vi "Save Rectifier Recipe.vi"(5 "Rev Mult":dbl format="%#_13g", 6 "Right AmpMins":dbl[](array[numeric]), 7 "Left AmpMins":dbl[](array[numeric]), 8 "error in":errorcluster, 9 "Number Steps":i32, 10 "Right Amps":dbl[](array[numeric]), 11 "Left Amps":dbl[](array[numeric])) -> (0 "error out":errorcluster, 2 "name":string, 3 "cancelled":bool)   [LabVIEW 2019]
uses:
  <vilib>/Utility/sysdir.llb/System Directory Type.ctl
  <vilib>/Utility/config.llb/Write Key (I32).vi
  <vilib>/Utility/config.llb/Write Key (Double).vi
  <vilib>/Utility/config.llb/NI_LVConfig.lvlib
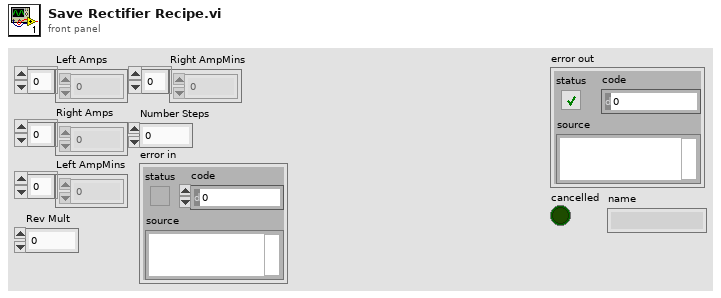
[diagram p1: front panel]
types:
  T1 = typedef "System Directory Type.ctl" = i32
  T2 = typedef "NI_LVConfig.lvlib/Config Data RefNum.ctl" = refnum<k1>
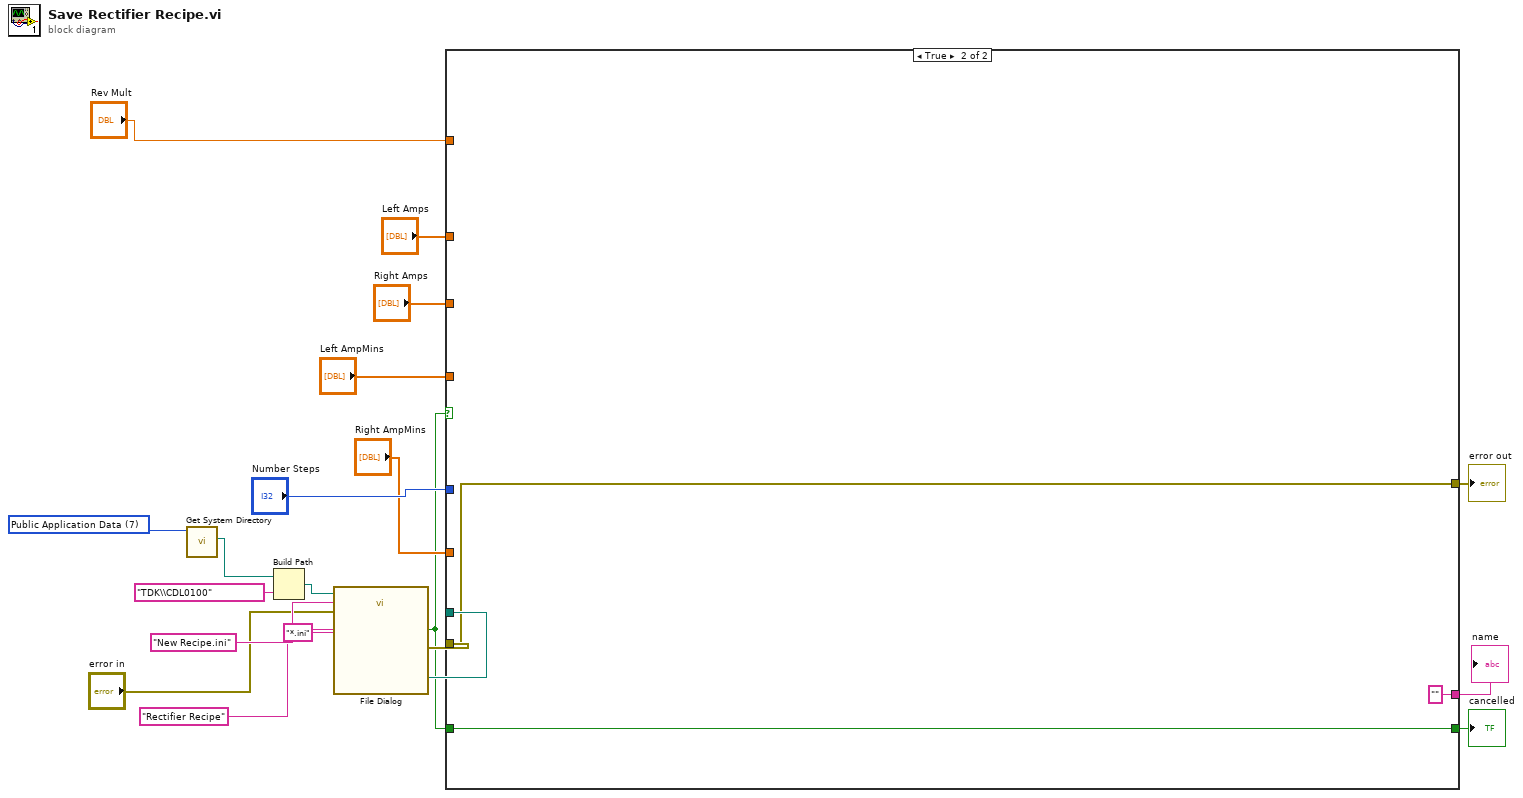
[diagram p0: block diagram]
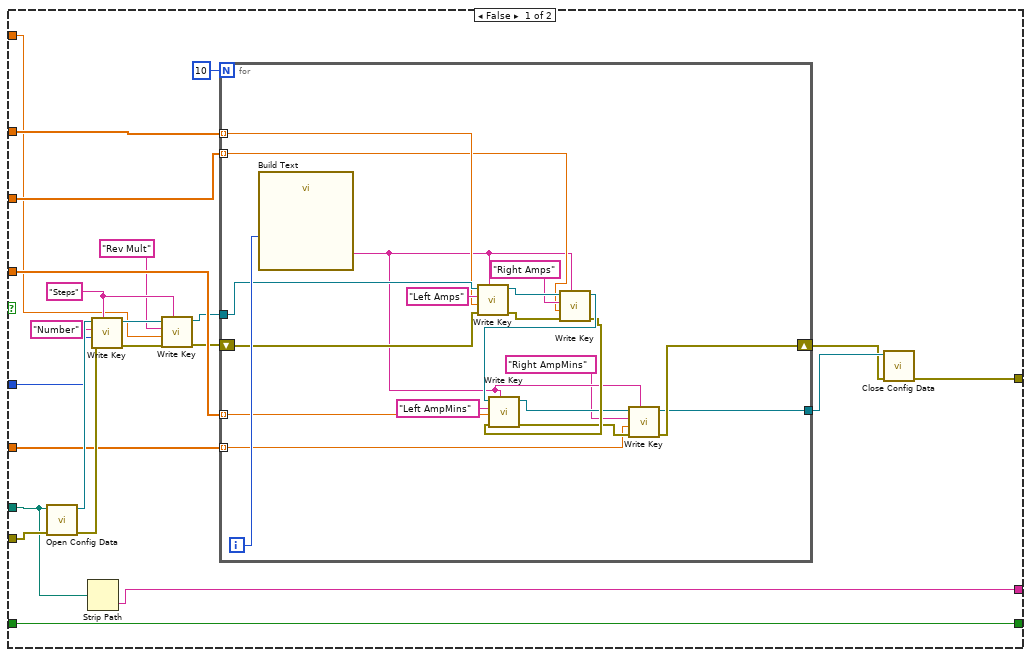
[diagram p2: hidden frame]
diagram:
  w20 = T1 7 items=["User Home"=0, "User Desktop"=1, "User Documents"=2, "User Application Data"=3, "User Preferences"=4, "User Temporary"=5, "Public Documents"=6, "Public Application Data"=7, "Public Preferences"=8, "Public Cache"=13, "System Core Libraries"=9, "System Installed Libraries"=10, "Application Files"=11, "Boot Volume Root"=12] ("system directory type")
  n1 = call <vilib>:"Get System Directory.vi"("system directory type"=w20) -> ("system directory"=w19:path)  [unwired: 10 in]
  n2 = Build Path(base path=w19, name or relative path="TDK\\CDL0100") -> (appended path=w17:path)
  n3 = call "File Dialog"("start path"=w17, "default name"="New Recipe.ini", "error in"="error in", "pattern (all files)"="*.ini", "pattern label"="Rectifier Recipe") -> ("selected path"=w12:path, "cancelled"=w3:bool, "error out"=w11:errorcluster)  [unwired: 7 in, 1 out]
  n4 = case shown="True" w3 {
    tunnel: w12 -> [w23 _]
    tunnel: w11 -> [w42 w66]
    tunnel: "Number Steps" -> [w39 _]
    tunnel: "Left Amps" -> [w37 _]
    tunnel: "Right Amps" -> [w36 _]
    tunnel: "Left AmpMins" -> [w35 _]
    tunnel: "Right AmpMins" -> [w34 _]
    tunnel: [w31 w66] -> w5
    tunnel: "Rev Mult" -> [w24 _]
    tunnel: w3 -> [w22 w65]
    tunnel: [w22 w65] -> w2
    tunnel: [w21 "" ("name")] -> w1
    frame False {
      w28 = "Steps" ("section")
      n5 = call <vilib>:"Open Config Data.vi"("error in (no error)"=w42, "configuration file path"=w23) -> ("error out"=w38:errorcluster, "refnum"=w41:T2)  [unwired: 7 in, 1 out]
      n6 = Strip Path(path=w23) -> (name=w21:string)  [unwired: 1 out]
      n7 = call-poly <vilib>:"Write Key.vi"("section"=w28, "error in (no error)"=w38, "value"=w39, "key"="Number", "refnum"=w41) -> ("error out"=w27:errorcluster, "refnum out"=w30:T2)  [unwired: 4 in, 1 out]
      n8 = call-poly <vilib>:"Write Key.vi"("section"=w28, "error in (no error)"=w27, "value"=w24, "key"="Rev Mult", "refnum"=w30) -> ("error out"=w26:errorcluster, "refnum out"=w29:T2)  [unwired: 4 in, 1 out]
      n9 = for {
        N: 10 -> [_]
        tunnel: w29 -> [w61]
        tunnel: w37 -> [w60] mode=indexing
        tunnel: w36 -> [w55] mode=indexing
        shift-right: [w48] -> w32
        shift-left: w26 -> [w59]
        tunnel: w35 -> [w51] mode=indexing
        tunnel: w34 -> [w45] mode=indexing
        tunnel: [w44] -> w33
        i -> [w62]
        n10 = call "Build Text"("d"=w62) -> ("Result"=w47:string)  [unwired: 13 in, 1 out]
        n11 = call-poly <vilib>:"Write Key.vi"("section"=w47, "error in (no error)"=w59, "value"=w60, "key"="Left Amps", "refnum"=w61) -> ("error out"=w56:errorcluster, "refnum out"=w58:T2)  [unwired: 4 in, 1 out]
        n12 = call-poly <vilib>:"Write Key.vi"("section"=w47, "error in (no error)"=w56, "value"=w55, "key"="Right Amps", "refnum"=w58) -> ("error out"=w53:errorcluster, "refnum out"=w54:T2)  [unwired: 4 in, 1 out]
        n13 = call-poly <vilib>:"Write Key.vi"("section"=w47, "error in (no error)"=w53, "value"=w51, "key"="Left AmpMins", "refnum"=w54) -> ("error out"=w49:errorcluster, "refnum out"=w50:T2)  [unwired: 4 in, 1 out]
        n14 = call-poly <vilib>:"Write Key.vi"("section"=w47, "error in (no error)"=w49, "value"=w45, "key"="Right AmpMins", "refnum"=w50) -> ("error out"=w48:errorcluster, "refnum out"=w44:T2)  [unwired: 4 in, 1 out]
      }
      n15 = call <vilib>:"Close Config Data.vi"("error in (no error)"=w32, "refnum"=w33) -> ("error out"=w31:errorcluster)  [unwired: 8 in, 1 out]
    }
    frame True {
    }
  }
  "error out" <- w5
  "cancelled" <- w2
  "name" <- w1
